vi "set up mmf aquisition.vi"(7 "inter-frame interval (ms)":dbl=200.0, 8 "error in (no error)":errorcluster, 11 "mmf path":path) -> (0 "error out":errorcluster, 1 "camera image is 8 bit":bool, 2 "camera image":T2, 3 "mmf parameters":T1={"mmf pointer"=0, "inter-frame interval (ms)"=200.0})   [LabVIEW 2021]
uses:
  <vilib>/vision/Image Controls.llb/IMAQ Image.ctl
  Image-Stack-Compressor/Stack Reader Wrapper/labview vis/StackReaderWrapper.lvlib
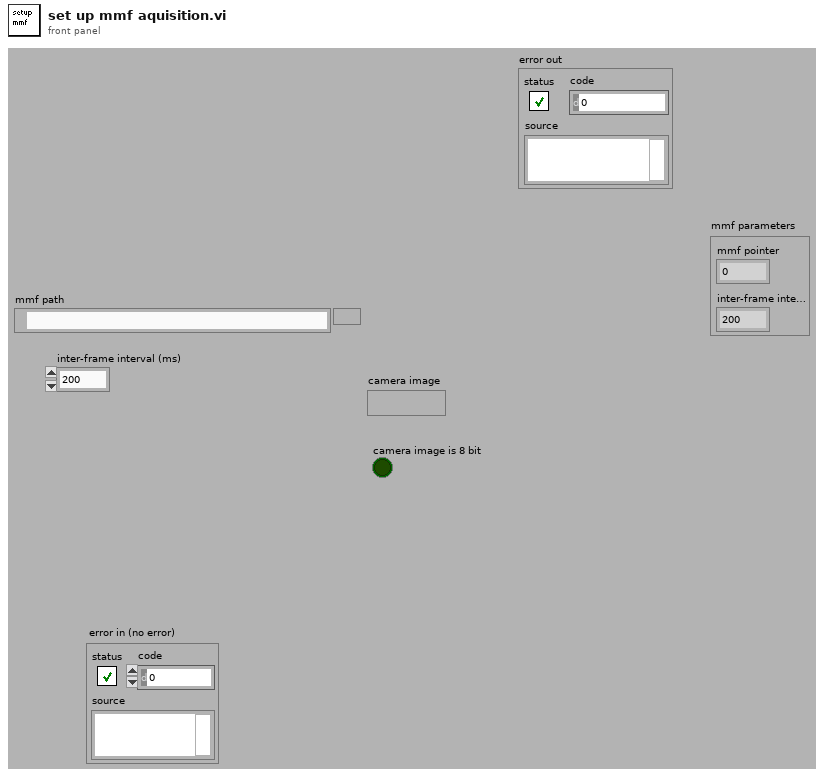
[diagram p1: front panel]
types:
  T1 = cluster{"mmf pointer":u32, "inter-frame interval (ms)":dbl}
  T2 = typedef "IMAQ Image.ctl" = refnum<image>
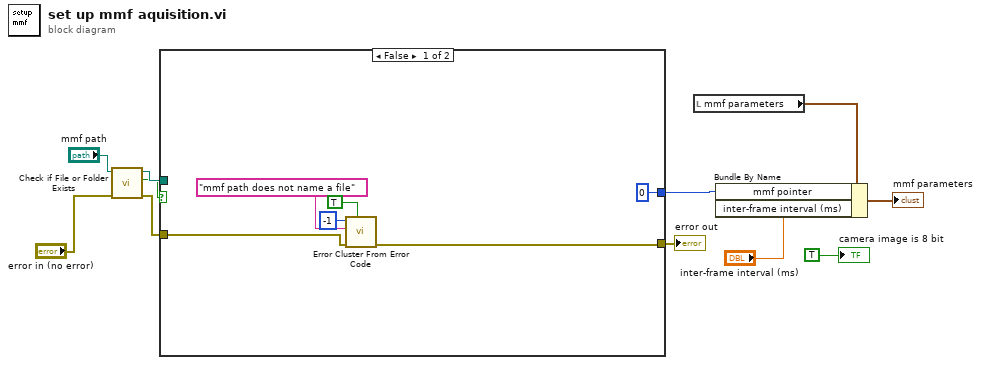
[diagram p0: block diagram]
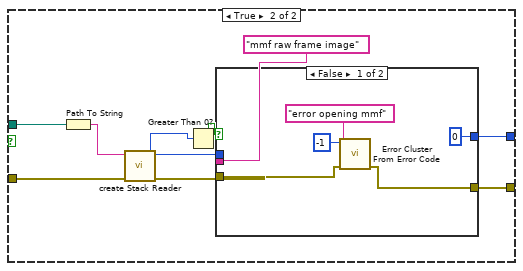
[diagram p2: hidden frame]
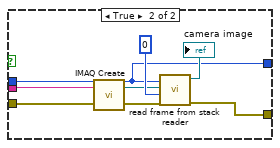
[diagram p3: hidden frame]
diagram:
  n1 = call <vilib>:"Check if File or Folder Exists.vi"("error in (no error)"="error in (no error)", "path"="mmf path") -> ("error out"=w8:errorcluster, "file or folder exists?"=w7:bool, "dup path"=w10:path)  [unwired: 7 in]
  n2 = case shown="False" w7 {
    tunnel: w10 -> [_ w23]
    tunnel: w8 -> [w17 w22]
    tunnel: [w15 w19] -> w5
    tunnel: [u32 0 ("function return") w18] -> w1
    frame False {
      n3 = call <vilib>:"Error Cluster From Error Code.vi"("show call chain? (False)"=TRUE, "error in (no error)"=w17, "error message (\"\")"="mmf path does not name a file" ("error message (\"\")"), "error code (0)"=-1) -> ("error out"=w15:errorcluster)  [unwired: 5 in]
    }
    frame True {
      n4 = Path To String(path=w23) -> (string=w25:string)
      n5 = call "create Stack Reader.vi"("error in (no error)"=w22, "fname"=w25) -> ("error out"=w24:errorcluster, "function return"=w20:u32)  [unwired: 8 in]
      n6 = Greater Than 0?(x=w20) -> (x > 0?=w21:bool)
      n7 = case shown="False" w21 {
        tunnel: "mmf raw frame image" ("Image Name") -> [_ w39]
        tunnel: w20 -> [_ w32]
        tunnel: w24 -> [w31 w36]
        tunnel: [w30 w34] -> w19
        tunnel: [u32 0 ("function return") w32] -> w18
        frame False {
          n8 = call <vilib>:"Error Cluster From Error Code.vi"("error in (no error)"=w31, "error message (\"\")"="error opening mmf" ("error message (\"\")"), "error code (0)"=-1) -> ("error out"=w30:errorcluster)  [unwired: 6 in]
        }
        frame True {
          n9 = call "IMAQ Create"("Image Name"=w39, "error in (no error)"=w36) -> ("New Image"=w37:T2, "error out"=w35:errorcluster)  [unwired: 3 in]
          n10 = call "read frame from stack reader.vi"("error in (no error)"=w35, "frameNumber"=0, "sr"=w32, "image dst"=w37) -> ("error out"=w34:errorcluster, "Image Out"=→"camera image":T2)  [unwired: 6 in]
        }
      }
    }
  }
  "error out" <- w5
  n11 = local read "mmf parameters"() -> (w3:T1)
  n12 = Bundle By Name(cluster=w3, "mmf pointer"=w1, "inter-frame interval (ms)"="inter-frame interval (ms)") -> (→"mmf parameters":T1)
  "camera image is 8 bit" <- TRUE ("camera image is 8 bit")
